vi "ExitLabVIEW_8.6.vi"   [LabVIEW 2014]
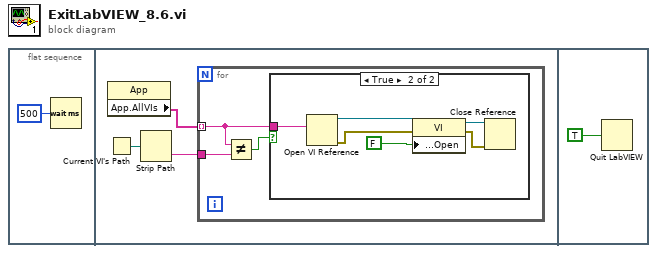
[diagram p0: block diagram]
diagram:
  n1 = flat-sequence {
    frame #0 {
      n2 = Wait (ms)(milliseconds to wait=u32 500) -> ()  [unwired: 1 out]
    }
    frame #1 {
      n3 = Current VI's Path() -> (path=w3:path)
      n4 = property class="App"() -> ("App.AllVIs"=w4:string[])  [unwired: 2 in, 2 out]
      n5 = Strip Path(path=w3) -> (name=w2:string)  [unwired: 1 out]
      n6 = for {
        tunnel: w4 -> [w6] mode=indexing
        tunnel: w2 -> [w5]
        n7 = Not Equal?(x=w6, y=w5) -> (x != y?=w7:bool)
        n8 = case shown="True" w7 {
          tunnel: w6 -> [_ w13]
          frame False {
          }
          frame True {
            n9 = Open VI Reference(vi path=w13) -> (vi reference=w9:refnum<vi>, error out=w8:errorcluster)  [unwired: 5 in]
            n10 = property class="VI"(reference=w9, error in=w8, "Front Panel.Open"=FALSE ("Front Panel Window:Open")) -> (reference out=w10:refnum<vi>, error out=w11:errorcluster)
            n11 = Close Reference(reference=w10, error in (no error)=w11) -> ()  [unwired: 1 out]
          }
        }
      }
    }
    frame #2 {
      n12 = Quit LabVIEW(quit? (T)=TRUE) -> ()
    }
  }
